vi "Image Dilate 2x2 (SubVI).vi"(0 "Data In":u8, 3 "Data Valid?":bool) -> (14 "Data Out":u8, 17 "Output Valid?":bool)   [LabVIEW 2015]
doc: "Filters input image and remove objects that are smaller than 128 x 128 pixels in size."
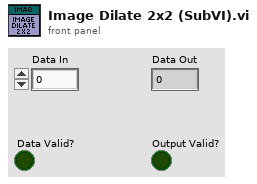
[diagram p1: front panel]
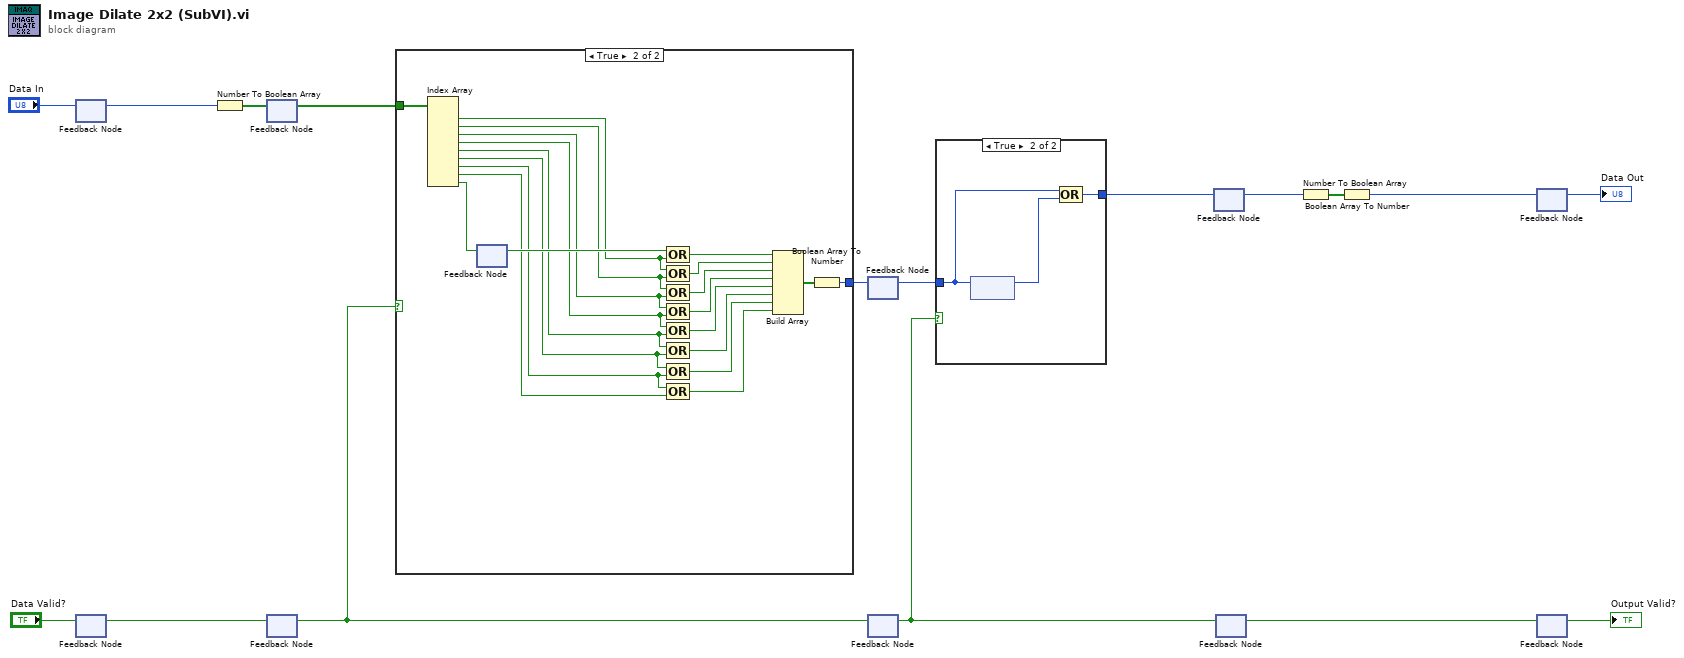
[diagram p0: block diagram]
diagram:
  n1 = feedback-in #1("Data In") -> ()
  n2 = feedback #1() -> (w6:u8)  [unwired: 1 in]
  n3 = feedback-in #2("Data Valid?") -> ()
  n4 = feedback #2() -> (w5:bool)  [unwired: 1 in]
  n5 = Number To Boolean Array(number=w6) -> (Boolean array=w10:bool[])
  n6 = feedback-in #3(w10) -> ()
  n7 = feedback #3() -> (w15:bool[])  [unwired: 1 in]
  n8 = feedback-in #4(w5) -> ()
  n9 = feedback #4() -> (w4:bool)  [unwired: 1 in]
  n10 = case shown="True" w4 {
    tunnel: [_ w26] -> w16
    tunnel: w15 -> [_ w25]
    frame False {
    }
    frame True {
      n11 = Index Array(array=w25) -> (element #1=w24:bool, element #2=w23:bool, element #3=w22:bool, element #4=w21:bool, element #5=w20:bool, element #6=w19:bool, element #7=w18:bool, element #8=w29:bool, element #9=w30:bool)  [unwired: 9 in]
      n12 = feedback #5() -> (w37:bool)  [unwired: 1 in]
      n13 = feedback-in #5(w30) -> ()
      n14 = Compound Arithmetic op=OR(w37, w24) -> (w38:bool)
      n15 = Compound Arithmetic op=OR(w24, w23) -> (w36:bool)
      n16 = Compound Arithmetic op=OR(w23, w22) -> (w35:bool)
      n17 = Compound Arithmetic op=OR(w22, w21) -> (w34:bool)
      n18 = Compound Arithmetic op=OR(w21, w20) -> (w33:bool)
      n19 = Compound Arithmetic op=OR(w20, w19) -> (w32:bool)
      n20 = Compound Arithmetic op=OR(w19, w18) -> (w31:bool)
      n21 = Compound Arithmetic op=OR(w18, w29) -> (w28:bool)
      n22 = Build Array(w38, w36, w35, w34, w33, w32, w31, w28) -> (w27:bool[])
      n23 = Boolean Array To Number(Boolean array=w27) -> (number=w26:u8)
    }
  }
  n24 = feedback-in #6(w16) -> ()
  n25 = feedback #6() -> (w12:u8)  [unwired: 1 in]
  n26 = feedback-in #7(w4) -> ()
  n27 = feedback #7() -> (w3:bool)  [unwired: 1 in]
  n28 = case shown="True" w3 {
    tunnel: [_ w41] -> w14
    tunnel: w12 -> [_ w40]
    frame False {
    }
    frame True {
      n29 = feedback #8() -> (w39:u8)  [unwired: 1 in]
      n30 = feedback-in #8(w40) -> ()
      n31 = Compound Arithmetic op=OR(w40, w39) -> (w41:u8)
    }
  }
  n32 = feedback-in #9(w14) -> ()
  n33 = feedback #9() -> (w17:u8)  [unwired: 1 in]
  n34 = feedback-in #10(w3) -> ()
  n35 = feedback #10() -> (w2:bool)  [unwired: 1 in]
  n36 = Number To Boolean Array(number=w17) -> (Boolean array=w1:bool[])
  n37 = Boolean Array To Number(Boolean array=w1) -> (number=w9:u8)
  n38 = feedback-in #11(w9) -> ()
  n39 = feedback #11() -> (→"Data Out":u8)  [unwired: 1 in]
  n40 = feedback-in #12(w2) -> ()
  n41 = feedback #12() -> (→"Output Valid?":bool)  [unwired: 1 in]
